vi "Actor Core.vi"(8 "error in":errorcluster, 11 "Measure Object in":refnum<class "Sweep Sequence.lvclass">) -> (0 "error out":errorcluster, 3 "Actor out":refnum<class "Actor.lvclass">)   [LabVIEW 2016, in "Sweep Sequence.lvclass"]
doc: "(<B>Filename</B>: Actor Framework.lvlib:Actor.lvclass:Actor Core.vi)\n\nReceives messages to the actor, reacts to them, and initiates any error handling that may shut the actor down.\n\nDescendant classes may override this VI to append parallel tasks for the actor to complete while it handles messages. Overrides use the Call Parent Method node."
uses:
  Sweep Sequence.lvclass
  C:/github/Measure_core/Da Base/Da Base.lvclass
  C:/Program Files/National Instruments/LabVIEW 2016/vi.lib/ActorFramework/Actor/Actor.lvclass
  <vilib>/ActorFramework/Actor/Actor.lvclass
  Sweep Sequence Configuration.ctl
  Da Base/Da Base.lvclass/Da Base.ctl
  <vilib>/ActorFramework/Actor/Actor.lvclass/Actor.ctl
  <vilib>/ActorFramework/Message Enqueuer/Message Enqueuer.lvclass/Message Enqueuer.ctl
  da Base/Read stop event.vi
  <vilib>/ActorFramework/Message Enqueuer/Init from Existing Queue.vi
  <vilib>/ActorFramework/Message Enqueuer/Enqueue.vi
  Da Base Messages/Configuration Value Changed Msg/Configuration Value Changed Msg.lvclass
  C:/Program Files/National Instruments/LabVIEW 2016/vi.lib/ActorFramework/Message/Message.lvclass
  <vilib>/ActorFramework/Message Priority Queue/Priority Enqueue.vi
  Sequence Element/Sequence Element.lvclass
  <vilib>/ActorFramework/Message Enqueuer/Message Enqueuer.lvclass
panel:
  in  "Configuration":T1 {"Duration" format="%#_6ps"}
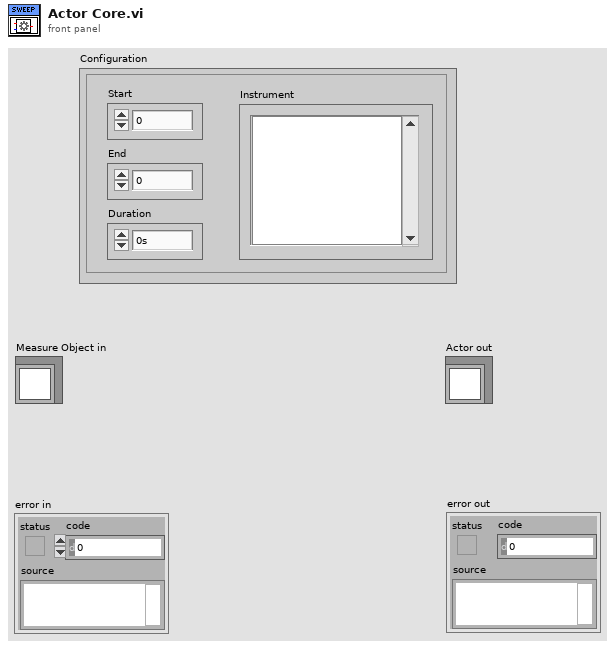
[diagram p1: front panel]
types:
  T1 = typedef "Sweep Sequence Configuration.ctl" = cluster{"Start":dbl, "End":dbl, "Duration":dbl, "Instrument":i32}
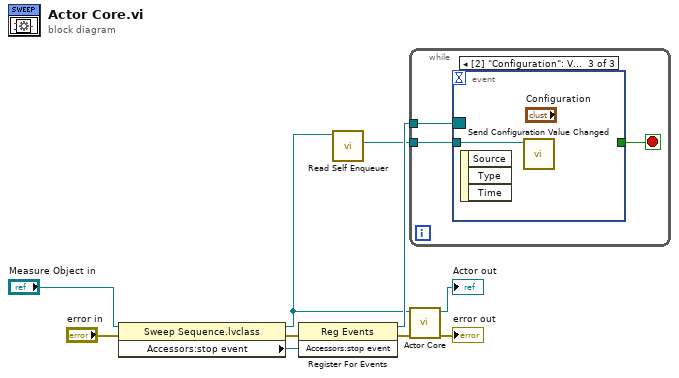
[diagram p0: block diagram]
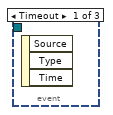
[diagram p2: hidden frame]
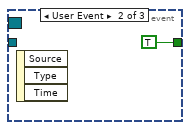
[diagram p3: hidden frame]
diagram:
  n1 = property class="Sweep Sequence.lvclass"(reference="Measure Object in", error in="error in") -> (reference out=w2:refnum<class "Sweep Sequence.lvclass">, error out=w7:errorcluster, "Accessors:stop event"=w4:refnum<user-event>)
  n2 = register-events(error in=w7, w4) -> (reference out=w3:refnum<event-registration>, error out=w5:errorcluster)  [unwired: 1 in]
  n3 = call <vilib>:"Read Self Enqueuer.vi"("Actor"=w2) -> ("Self Enqueuer"=w1:refnum<class "Message Enqueuer.lvclass">)  [unwired: 10 in]
  n4 = while {
    tunnel: w3 -> [w13]
    tunnel: w1 -> [w11]
    stop <- w12 stop-if-true
    n5 = event shown="[2] \"Configuration\": Value Change" {
      selector: w13 -> [_ _ _]
      dyn-events: _ -> [_ _ _]
      timeout: _ -> [_ _ _]
      tunnel: [_ TRUE _] -> w12
      tunnel: w11 -> [_ _ w15]
      event Timeout {
        n6 = event-data() -> ()  [unwired: 1 in, 3 out]
      }
      event User Event {
        n7 = event-data() -> ()  [unwired: 1 in, 3 out]
      }
      event Value Change {
        n8 = event-data() -> ()  [unwired: 1 in, 3 out]
        n9 = call "Send Configuration Value Changed.vi"("Message Enqueuer"=w15) -> ()  [unwired: 9 in, 2 out]
      }
    }
  }
  n10 = call-parent "Actor Core.vi"("error in"=w5, "Measure Object in"=w2) -> ("error out"=→"error out":errorcluster, "Actor out"=→"Actor out":refnum<class "Actor.lvclass">)  [unwired: 8 in]
